vi "Keithley 2002 Disp2 Config.vi"(1 "error in":T1, 2 "display (off:0)":u16(ring) items=["off", "previous", "next"], 3 "GPIB address":string="16") -> (0 "error out":T1)   [LabVIEW 2020]
doc: "This VI is used to configure the secondary display settings.\n\nThis includes secondary functions that aren't normally performed each time a measurement is taken.\n\nTo read the secondary display, use the Disp2 Read VI."
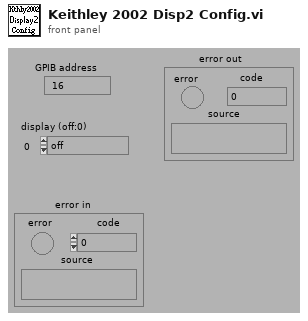
[diagram p1: front panel]
types:
  T1 = cluster{"error":bool, "code":i32, "source":string}
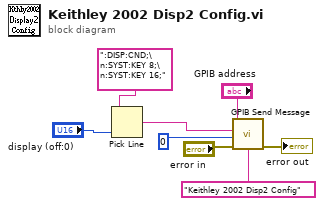
[diagram p0: block diagram]
diagram:
  n1 = Pick Line(multi-line string=":DISP:CND;\n:SYST:KEY 8;\n:SYST:KEY 16;", line index="display (off:0)") -> (output string=w5:string)  [unwired: 1 in]
  n2 = call "GPIB Send Message.vi"("address string"="GPIB address", "write buffer"=w5, "source"="Keithley 2002 Disp2 Config", "write mode (set END:0)"=0, "error in"="error in") -> ("error out"=→"error out":T1)  [unwired: 2 in, 2 out]
